vi "Remove Comments.vi"(8 "error in (no error)":errorcluster, 11 "String":string) -> (0 "error out":errorcluster, 3 "string":string)   [LabVIEW 2019]
uses:
  <userlib>/_OpenG.lib/array/array.llb/Filter 1D Array (U8)__ogtk.vi
  <userlib>/NEVSTOP-Programming-Palette/Configuration/Ini/ini_configuration.lvlib
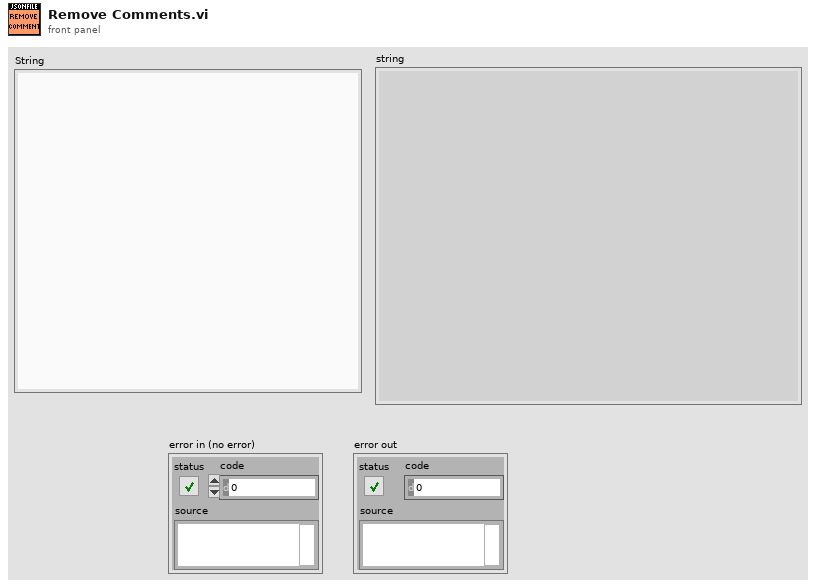
[diagram p1: front panel]
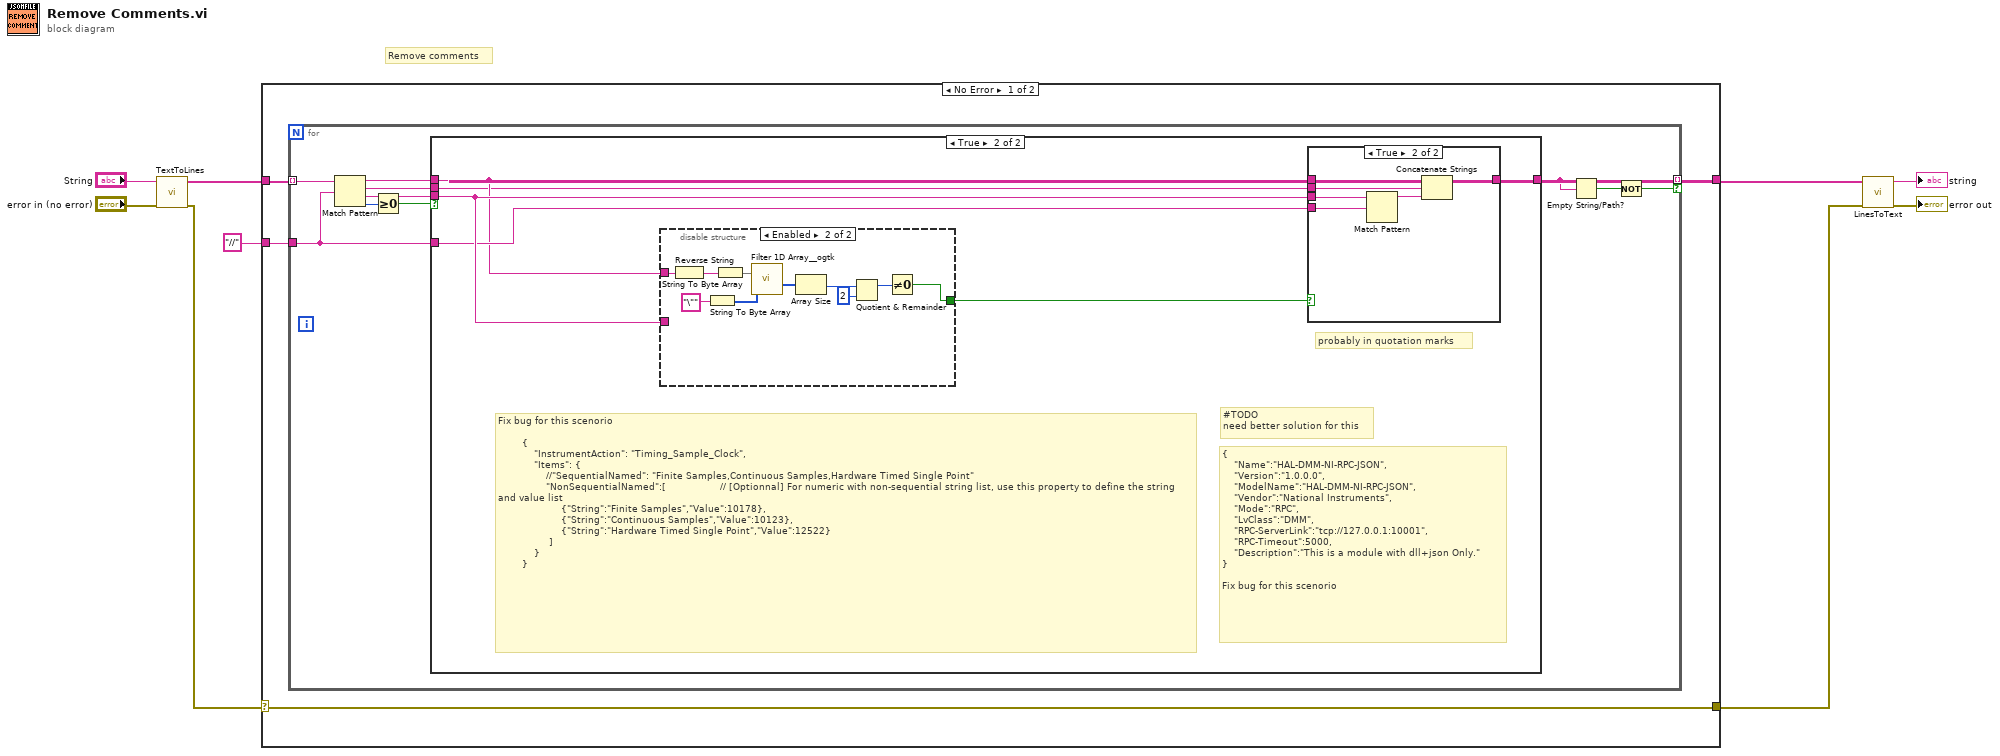
[diagram p0: block diagram]
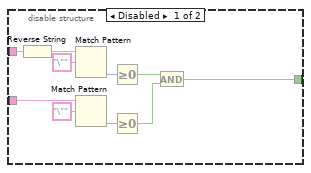
[diagram p3: hidden frame]
diagram:
  # "Remove comments"
  n1 = call <userlib>:"TextToLines.vi"("error in (no error)"="error in (no error)", "string"="String") -> ("error out"=w3:errorcluster, "Lines"=w2:string[])  [unwired: 8 in]
  n2 = case shown="No Error" w3 {
    selector: w3 -> [w11 w58]
    tunnel: [w11 w58] -> w5
    tunnel: w2 -> [w13 _]
    tunnel: [w12 _] -> w4
    tunnel: "//" ("Annotation Seperator(#)") -> [w10 _]
    frame No Error {
      n3 = for {
        tunnel: w13 -> [w22] mode=indexing
        tunnel: [w17] -> w12 mode=indexing if=w23
        tunnel: w10 -> [w14]
        n4 = Match Pattern(string=w22, regular expression=w14) -> (before substring=w18:string, match substring=w15:string, after substring=w16:string, offset past match=w20:i32)  [unwired: 1 in]
        n5 = Greater Or Equal To 0?(x=w20) -> (x >= 0?=w19:bool)
        n6 = case shown="True" w19 {
          tunnel: w18 -> [w24 w28]
          tunnel: [w24 w26] -> w17
          tunnel: w16 -> [_ w30]
          tunnel: w15 -> [_ w27]
          tunnel: w14 -> [_ w29]
          frame False {
          }
          frame True {
            # "Fix bug for this scenorio\n\n        {\n            \"InstrumentAction\": \"Timing_Sample_Clock\",\n            \"Items\": {\n                //\"SequentialNamed\": \"Finite Samples,Continuous Samples,Hardware Timed Single Point\"\n                \"NonSequentialNamed\":[                  // [Optionnal] For numeric with non-sequential string list, use this property to define the string and value list\n                     {\"String\":\"Finite Samples\",\"Value\":10178},\n                     {\"String\":\"Continuous Samples\",\"Value\":10123},\n                     {\"String\":\"Hardware Timed Single Point\",\"Value\":12522}\n                 ]\n            }\n        }"
            # "#TODO\nneed better solution for this"
            # "{\n    \"Name\":\"HAL-DMM-NI-RPC-JSON\",\n    \"Version\":\"1.0.0.0\",\n    \"ModelName\":\"HAL-DMM-NI-RPC-JSON\",\n    \"Vendor\":\"National Instruments\",\n    \"Mode\":\"RPC\",\n    \"LvClass\":\"DMM\",\n    \"RPC-ServerLink\":\"tcp://127.0.0.1:10001\",\n    \"RPC-Timeout\":5000,\n    \"Description\":\"This is a module with dll+json Only.\"\n}\n\nFix bug for this scenorio"
            # "probably in quotation marks"
            n7 = disable-structure shown="Enabled" {
              disable-tunnel: w30 -> [w33 _]
              disable-tunnel: w28 -> [w32 w50]
              disable-tunnel: [w31 w41] -> w25
              frame Disabled {
                n8 = Reverse String(1:w32) -> (0:w40:string)
                n9 = Match Pattern(string=w40, regular expression="\"") -> (offset past match=w37:i32)  [unwired: 1 in, 3 out]
                n10 = Match Pattern(string=w33, regular expression="\"") -> (offset past match=w36:i32)  [unwired: 1 in, 3 out]
                n11 = Greater Or Equal To 0?(x=w37) -> (x >= 0?=w35:bool)
                n12 = Greater Or Equal To 0?(x=w36) -> (x >= 0?=w34:bool)
                n13 = And(x=w35, y=w34) -> (x .and. y?=w31:bool)
              }
              frame Enabled {
                n14 = Reverse String(1:w50) -> (0:w48:string)
                n15 = String To Byte Array(string="\"" ("regular expression")) -> (unsigned byte array=w46:u8[])
                n16 = String To Byte Array(string=w48) -> (unsigned byte array=w49:u8[])
                n17 = call-poly <userlib>:"Filter 1D Array__ogtk.vi"("items to filter"=w46, "array"=w49) -> ("filtered item indices"=w45:i32[])  [unwired: 4 in, 1 out]
                n18 = Array Size(array=w45) -> (size(s)=w44:i32)
                n19 = Quotient & Remainder(x=w44, y=2) -> (x-y*floor(x/y)=w42:i32)  [unwired: 1 out]
                n20 = Not Equal To 0?(x=w42) -> (x != 0?=w41:bool)
              }
            }
            n21 = case shown="True" w25 {
              tunnel: w30 -> [_ w57]
              tunnel: w29 -> [_ w56]
              tunnel: w28 -> [w51 w55]
              tunnel: w27 -> [_ w54]
              tunnel: [w51 w52] -> w26
              frame False {
              }
              frame True {
                n22 = Match Pattern(string=w57, regular expression=w56) -> (before substring=w53:string)  [unwired: 1 in, 3 out]
                n23 = Concatenate Strings(w55, w54, w53) -> (w52:string)
              }
            }
          }
        }
        n24 = Empty String/Path?(string/path=w17) -> (empty?=w21:bool)
        n25 = Not(x=w21) -> (.not. x?=w23:bool)
      }
    }
    frame Error {
    }
  }
  n26 = call <userlib>:"LinesToText.vi"("error in (no error)"=w5, "Lines"=w4) -> ("error out"=→"error out":errorcluster, "string"=→"string":string)  [unwired: 8 in]
